vi "movingAverage(SubVI).vi"(10 "length":i32, 11 "all rows":dbl[](array[numeric])) -> (3 "Array":dbl[](array[numeric]))   [LabVIEW 2019]
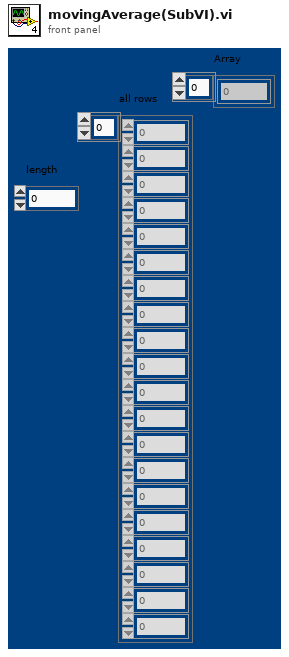
[diagram p1: front panel]
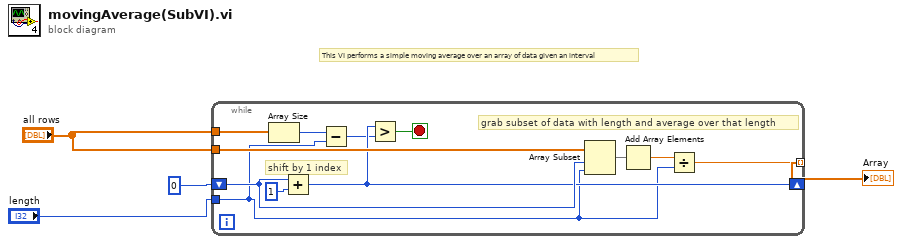
[diagram p0: block diagram]
diagram:
  # "This VI performs a simple moving average over an array of data given an interval"
  n1 = while {
    tunnel: "all rows" -> [w14]
    shift-right: [w10] -> _
    shift-left: 0 ("index") -> [w13]
    tunnel: "length" -> [w7]
    tunnel: [w11] -> w3 mode=indexing
    tunnel: "all rows" -> [w8]
    stop <- w9 stop-if-true
    # "grab subset of data with length and average over that length"
    # "shift by 1 index"
    n2 = Array Size(array=w8) -> (size(s)=w6:i32)
    n3 = Add(x=w13, y=1) -> (x+y=w10:i32)
    n4 = Subtract(x=w6, y=w7) -> (x-y=w5:i32)
    n5 = Greater?(x=w10, y=w5) -> (0:w9:bool)
    n6 = Array Subset(array=w14, index=w13, length=w7) -> (w15:dbl[])
    n7 = Add Array Elements(numeric array=w15) -> (sum=w16:dbl)
    n8 = Divide(x=w16, y=w7) -> (x/y=w11:dbl)
  }
  "Array" <- w3
